vi "json Parse Boolean - string path.vi"(8 "error in (no error)":errorcluster, 9 "default":bool, 10 "path":string, 11 "JSON Document in":refnum<class "JSON Document.lvclass">) -> (0 "error out":errorcluster, 1 "defaulted?":bool, 2 "value":bool, 3 "JSON Document out":refnum<class "JSON Document.lvclass">)   [LabVIEW 2015, in "JSON Document.lvclass"]
uses:
  JSON Document.lvclass
  JSON Document.lvclass/JSON Document.ctl
  rapidjson wrapper/rapidjson wrapper.lvlib
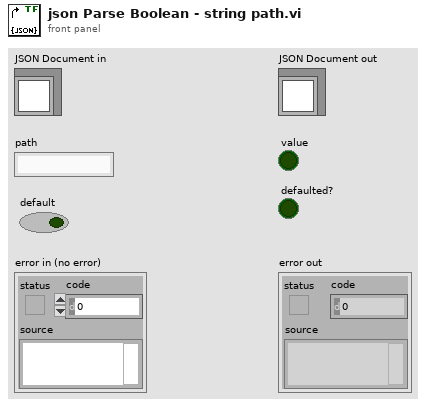
[diagram p1: front panel]
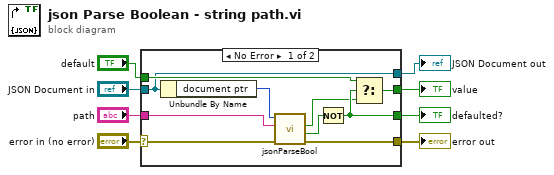
[diagram p0: block diagram]
diagram:
  n1 = case shown="No Error" "error in (no error)" {
    selector: "error in (no error)" -> [w18 w21]
    tunnel: [w15 w21] -> w7
    tunnel: [w14 w20] -> w5
    tunnel: "JSON Document in" -> [w14 w20]
    tunnel: "default" -> [w16 w19]
    tunnel: "path" -> [w12 _]
    tunnel: [w17 w19] -> w2
    tunnel: [w13 _] -> w1
    frame No Error {
      n2 = Unbundle By Name(w14) -> ("document ptr"=w11:i64)
      n3 = call "jsonParseBool.vi"("error in (no error)"=w18, "path"=w12, "d in"=w11) -> ("error out"=w15:errorcluster, "sucess?"=w10:bool, "value"=w9:bool)  [unwired: 5 in, 1 out]
      n4 = Not(x=w10) -> (.not. x?=w13:bool)
      n5 = Select(t=w16, s=w13, f=w9) -> (s? t:f=w17:bool)
    }
    frame Error {
    }
  }
  "error out" <- w7
  "JSON Document out" <- w5
  "value" <- w2
  "defaulted?" <- w1
